vi "ClearDAQmxTasks_All.vi"   [LabVIEW 2022 SP3]
uses:
  <resource>/objmgr/daqmx.rc
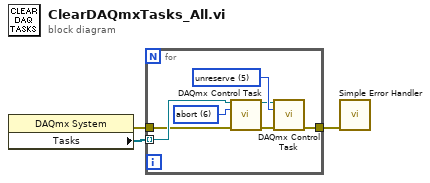
[diagram p0: block diagram]
diagram:
  n1 = property class="DAQmx System"() -> (error out=w2:errorcluster, "Tasks"=w3:refnum<k21>[])  [unwired: 2 in, 1 out]
  n2 = for {
    tunnel: w3 -> [w7] mode=indexing
    tunnel: w2 -> [w6]
    tunnel: [w4] -> w1
    w9 = 5 items=["verify"=2, "reserve"=4, "commit"=3, "unreserve"=5, "abort"=6] ("action")
    w10 = 6 items=["verify"=2, "reserve"=4, "commit"=3, "unreserve"=5, "abort"=6] ("action")
    n3 = call <vilib>:"DAQmx Control Task.vi"("task/channels in"=w7, "action"=w10, "error in"=w6) -> ("task out"=w8:refnum<k21>, "error out"=w5:errorcluster)  [unwired: 11 in]
    n4 = call <vilib>:"DAQmx Control Task.vi"("task/channels in"=w8, "action"=w9, "error in"=w5) -> ("error out"=w4:errorcluster)  [unwired: 11 in, 1 out]
  }
  n5 = call <vilib>:"Simple Error Handler.vi"("error in (no error)"=w1) -> ()  [unwired: 4 in, 5 out]
